vi "SQL-清空数据库信息.vi"(8 "error in (no error)":errorcluster caption="错误输入（无错误）", 10 "字符串":string) -> (0 "error out":errorcluster caption="错误输出")   [LabVIEW 2017]
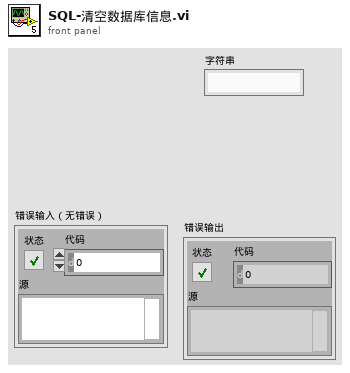
[diagram p1: front panel]
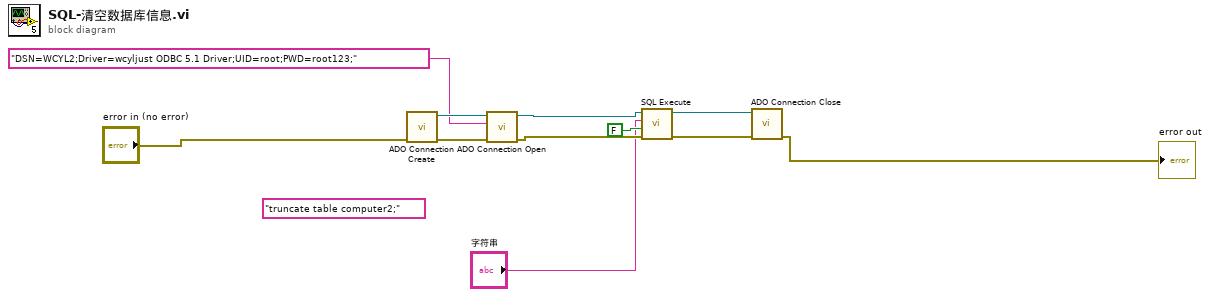
[diagram p0: block diagram]
diagram:
  (unwired) "truncate table computer2;" ("Command Text")
  n1 = call <userlib>:"ADO Connection Create.vi"("error in (no error)"="error in (no error)") -> ("error out"=w9:errorcluster, "ADODB._Connection Out"=w10:refnum<k7>)  [unwired: 9 in]
  n2 = call <userlib>:"ADO Connection Open.vi"("error in (no error)"=w9, "ConnectionString"="DSN=WCYL2;Driver=wcyljust ODBC 5.1 Driver;UID=root;PWD=root123;", "ADODB._Connection In"=w10) -> ("error out"=w2:errorcluster, "ADODB._Connection Out"=w3:refnum<k7>)  [unwired: 7 in]
  n3 = call <userlib>:"SQL Execute.vi"("error in (no error)"=w2, "Return Data (T)"=FALSE, "Command Text"="字符串", "ADODB._Connection In"=w3) -> ("error out"=w6:errorcluster, "ADODB._Connection Out"=w7:refnum<k7>)  [unwired: 4 in, 2 out]
  n4 = call <userlib>:"ADO Connection Close.vi"("error in (no error)"=w6, "ADODB._Connection In"=w7) -> ("error out"=→"error out":errorcluster)  [unwired: 8 in, 1 out]
